vi "PID EGU to Percentage (DBL Array).vi"(1 "minimum (EGU)":dbl[](array[numeric])=[0.0] format="%.2f", 2 "input (EGU)":dbl[](array[numeric])=[0.0] format="%.2f", 3 "maximum (EGU)":dbl[](array[numeric])=[0.0] format="%.2f") -> (0 "% span":dbl[](array[numeric]) format="%.2f")   [LabVIEW 2017, in "NI_PID_pid.lvlib"]
doc: "Converts an engineering-units input to a percent-of-range output based on the minimum and maximum range settings. Use the DBL instance of this VI to implement a single control loop. Use the DBL Array instance to implement parallel multi-loop control."
uses:
  <vilib>/addons/control/pid/NI_PID_pid.lvlib
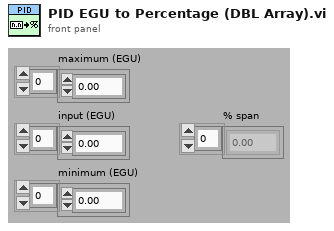
[diagram p1: front panel]
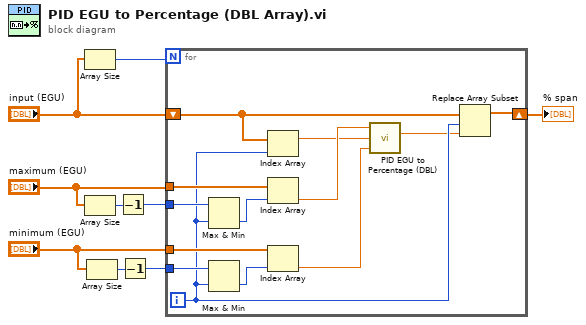
[diagram p0: block diagram]
diagram:
  n1 = Array Size(array="input (EGU)") -> (size(s)=w1:i32)
  n2 = Array Size(array="maximum (EGU)") -> (size(s)=w6:i32)
  n3 = Array Size(array="minimum (EGU)") -> (size(s)=w3:i32)
  n4 = Decrement(x=w6) -> (x-1=w5:i32)
  n5 = Decrement(x=w3) -> (x-1=w2:i32)
  n6 = for {
    N: w1 -> [_]
    tunnel: "maximum (EGU)" -> [w19]
    tunnel: "minimum (EGU)" -> [w20]
    shift-right: [w21] -> w8
    shift-left: "input (EGU)" -> [w22]
    tunnel: w5 -> [w18]
    tunnel: w2 -> [w17]
    i -> [w14]
    n7 = Max & Min(x=w18, y=w14) -> (min(x,y)=w15:i32)  [unwired: 1 out]
    n8 = Max & Min(x=w17, y=w14) -> (min(x,y)=w16:i32)  [unwired: 1 out]
    n9 = Index Array(array=w22, index=w14) -> (element=w12:dbl)
    n10 = Index Array(array=w19, index=w15) -> (element=w13:dbl)
    n11 = Index Array(array=w20, index=w16) -> (element=w11:dbl)
    n12 = call <vilib>:"PID EGU to Percentage (DBL).vi"("minimum (EGU)"=w11, "input (EGU)"=w12, "maximum (EGU)"=w13) -> ("% span"=w10:dbl)
    n13 = Replace Array Subset(array=w22, new element=w10, index=w14) -> (w21:dbl[])
  }
  "% span" <- w8
